vi "Get Keywords.vi"(8 "error in (no error)":errorcluster, 11 "Structure Loop in":refnum<class "Structure Loop.lvclass">) -> (0 "error out":errorcluster, 2 "Keywords":string[](array[string]), 3 "Structure Loop out":refnum<class "Structure Loop.lvclass">)   [LabVIEW 2019, in "Structure Loop.lvclass"]
uses:
  Structure Loop.lvclass
  functionsbase/functionbase.lvclass
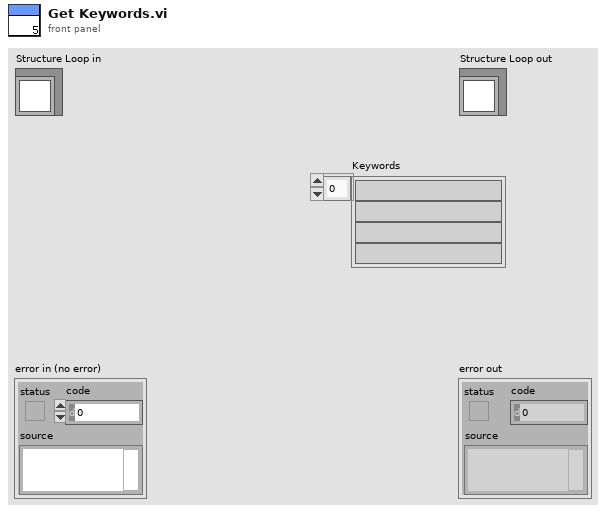
[diagram p1: front panel]
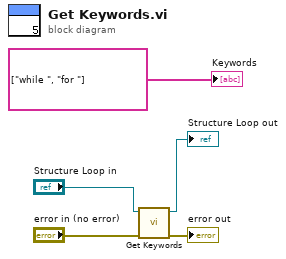
[diagram p0: block diagram]
diagram:
  n1 = call-parent "Get Keywords.vi"("error in (no error)"="error in (no error)", "functionbase in"="Structure Loop in") -> ("error out"=→"error out":errorcluster, "functionbase out"=→"Structure Loop out":refnum<class "Structure Loop.lvclass">)  [unwired: 7 in, 1 out]
  "Keywords" <- string[] ["while ", "for "] ("Keywords")
